vi "PathPlanner_TrajectoryState_GetAll.vi"(11 "PathPlannerState":T4={"TimeSeconds"=0.0, "VelocityMPS"=0.0, "AccerationMpsSq"=0.0, "HeadingAngularVelRadPerSec"=0.0, "PositionMeters"={"X"=0.0, "Y"=1.0}, "Heading"={"VALUE"=0.0, "COS"=1.0, "SIN"=0.0}, "TargetHolonomicRotation"={"VALUE"=0.0, "COS"=1.0, "SIN"=0.0}, "CurvatureRadPerMeter"=0.0, "DeltaPos"=0.0, "PathPlannerConstraints"={"MaxVelocityMps;"=0.0, "MaxAccelerationMpsSq;"=0.0, "MaxAngularVelRadPsEc;"=0.0, "MaxAngularAccRadPSecSq"=0.0}} {"TargetHolonomicRotation"."SIN" format="%13.4f"; "TargetHolonomicRotation"."COS" format="%13.4f"; "TargetHolonomicRotation"."VALUE" format="%13.4f"; "Heading"."SIN" format="%13.4f"; "Heading"."COS" format="%13.4f"; "Heading"."VALUE" format="%13.4f"; "PositionMeters"."Y" format="%14.3f"; "PositionMeters"."X" format="%14.3f"}) -> (0 "Heading":T2={"VALUE"=0.0, "COS"=1.0, "SIN"=0.0} {"SIN" format="%13.4f"; "COS" format="%13.4f"; "VALUE" format="%13.4f"}, 1 "PositionMeters":T3 {"Y" format="%14.3f"; "X" format="%14.3f"}, 2 "HeadingAngularVelRadPerSec":dbl, 3 "AccerationMpsSq":dbl, 4 "TargetHolonomicRotation":T2={"VALUE"=0.0, "COS"=1.0, "SIN"=0.0} {"SIN" format="%13.4f"; "COS" format="%13.4f"; "VALUE" format="%13.4f"}, 5 "VelocityMPS":dbl, 6 "CurvatureRadPerMeter":dbl, 7 "TimeSeconds":dbl, 8 "PathPlannerConstraints":T1)   [LabVIEW 2019, in "PathPlanner24.lvlib"]
doc: "Create a trajectory state\n\nInputs:\n -- timeSeconds - double - The time at this state in seconds ( default = 0; )\n -- velocityMps - double - The velocity at this state in m/s ( default = 0 )\n -- accelerationMpsSq - double - The acceleration at this state in m/s^2 ( default = 0 )\n -- headingAngularVelocityRps - double - The time at this state in seconds ( default = 0 )\n -- positionMeters - translation2d - The position at this state in meters ( default = 0,0 )\n -- heading - rotation2d - The heading (direction of travel) at this state ( default = 0 )\n -- targetHolonomicRotation - rotation2d - The target holonomic rotation at this state ( default = 0 )\n -- curvatureRadPerMeter - double - The curvature at this state in rad/m ( default = 0 )\n -- constraints -- cluster -- constraints to apply at this state (default - none )\n\n\nOutputs\n - PathPlannerTrajectoryState -- cluster -- Newly created state"
uses:
  PathPlanner24.lvlib
  <vilib>/Rock Robotics/WPI/ThirdParty/JAS_Junk/TrajLib/TypeDef/ROTATION2D.ctl
  <vilib>/Rock Robotics/WPI/ThirdParty/JAS_Junk/TrajLib/Trajectory_Library.lvlib
  <vilib>/Rock Robotics/WPI/ThirdParty/JAS_Junk/TrajLib/TypeDef/TRANSLATION2D.ctl
  TypeDef/PathPlannerTrajectoryState.ctl
  TypeDef/PathPlannerPathConstraints.ctl
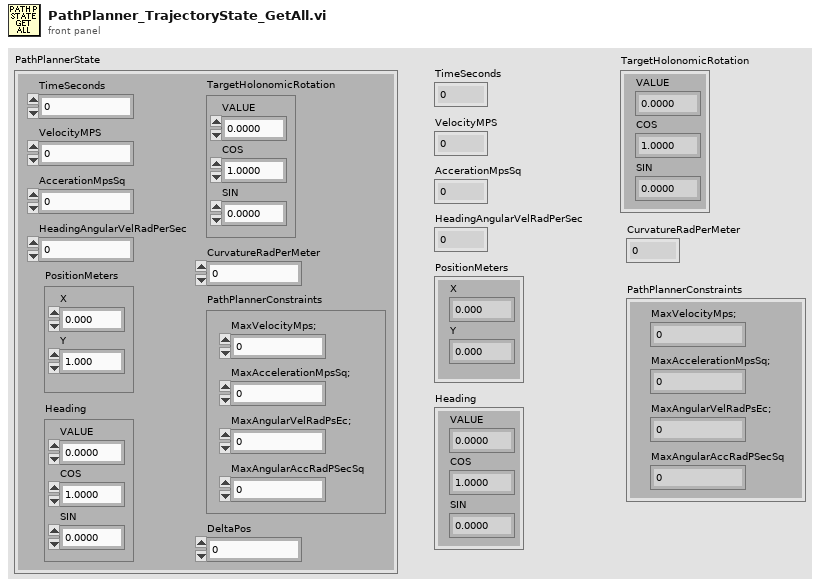
[diagram p1: front panel]
types:
  T1 = typedef "PathPlanner24.lvlib/PathPlannerPathConstraints.ctl" = cluster{"MaxVelocityMps;":dbl, "MaxAccelerationMpsSq;":dbl, "MaxAngularVelRadPsEc;":dbl, "MaxAngularAccRadPSecSq":dbl}
  T2 = typedef "Trajectory_Library.lvlib/ROTATION2D.ctl" = cluster{"VALUE":dbl, "COS":dbl, "SIN":dbl}
  T3 = typedef "Trajectory_Library.lvlib/TRANSLATION2D.ctl" = cluster{"X":dbl, "Y":dbl}
  T4 = typedef "PathPlanner24.lvlib/PathPlannerTrajectoryState.ctl" = cluster{"TimeSeconds":dbl, "VelocityMPS":dbl, "AccerationMpsSq":dbl, "HeadingAngularVelRadPerSec":dbl, "PositionMeters":T3, "Heading":T2, "TargetHolonomicRotation":T2, "CurvatureRadPerMeter":dbl, "DeltaPos":dbl, "PathPlannerConstraints":T1}
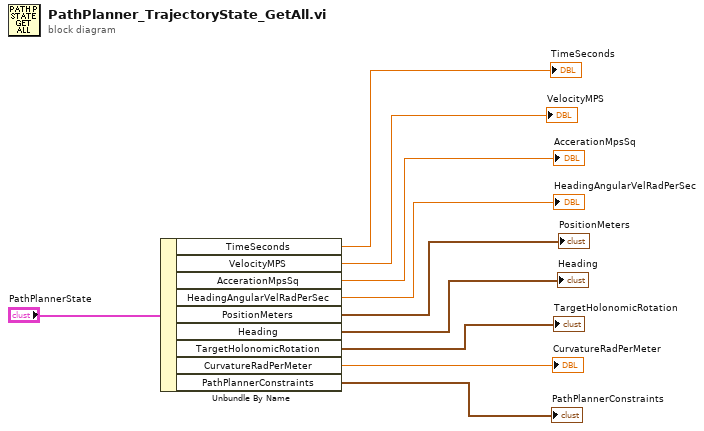
[diagram p0: block diagram]
diagram:
  n1 = Unbundle By Name("PathPlannerState") -> ("TimeSeconds"=→"TimeSeconds":dbl, "VelocityMPS"=→"VelocityMPS":dbl, "AccerationMpsSq"=→"AccerationMpsSq":dbl, "HeadingAngularVelRadPerSec"=→"HeadingAngularVelRadPerSec":dbl, "PositionMeters"=→"PositionMeters":T3, "Heading"=→"Heading":T2, "TargetHolonomicRotation"=→"TargetHolonomicRotation":T2, "CurvatureRadPerMeter"=→"CurvatureRadPerMeter":dbl, "PathPlannerConstraints"=→"PathPlannerConstraints":T1)
